vi "test main.vi"(8 "error in (no error)":errorcluster) -> (0 "error out":errorcluster)   [LabVIEW 2023]
uses:
  sequenceManagerWorker/sequenceManagerWorker.lvclass
  sequenceManagerWorker/ZE_Easy.Sequencer.lvlibp/Step/Step.lvclass
  f0be651f-cbc1-426a-b5fe-e5e117e5ce35.vi
  f17cfda4-eca7-44fe-abc0-9ba8470d04ab.vi
  ee86c54d-6899-49db-a6a4-df2ffb5378ed.vi
  d3de8112-106e-4eb0-9e2c-686bfc4be21a.vi
  7af16d0e-3bb2-44d1-b501-a320892e61ce.vi
  <vilib>/addons/_JKI Toolkits/Caraya/classes/Assert/Assert Equal Value and Type_Variant.vi
  <vilib>/addons/_JKI Toolkits/Caraya/classes/Assert/Assert Not Error.vi
  sequenceManagerWorker/ZE_Easy.Sequencer.lvlibp/Parameter/Parameter.lvclass
  <vilib>/addons/_JKI Toolkits/Caraya/classes/Test/Test.lvclass
  <vilib>/addons/_JKI Toolkits/Caraya/classes/Assert/Assert.lvclass
panel:
  # "Connector Pane"
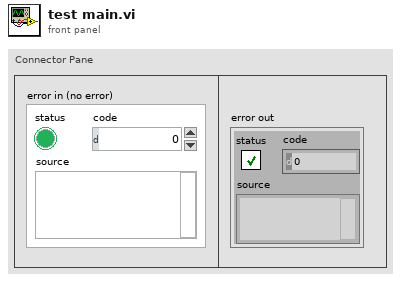
[diagram p1: front panel]
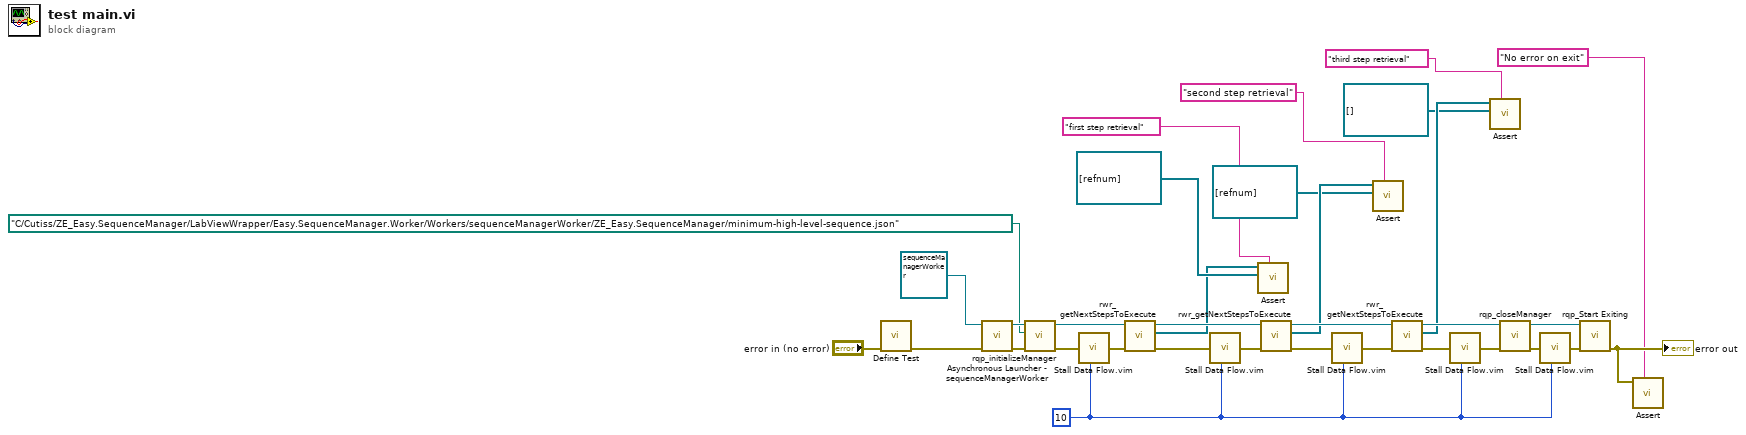
[diagram p0: block diagram]
diagram:
  w1 = u32 10 ("milliseconds to wait")
  n1 = call <vilib>:"Define Test.vi"("error in (no error)"="error in (no error)") -> ("error out"=w15:errorcluster)  [unwired: 9 in, 1 out]
  n2 = call "Asynchronous Launcher - sequenceManagerWorker.vi"("error in"=w15, "sequenceManagerWorker in"=refnum<class "sequenceManagerWorker.lvclass"> refnum) -> ("error out"=w31:errorcluster, "sequenceManagerWorker out"=w32:refnum<class "sequenceManagerWorker.lvclass">)  [unwired: 8 in]
  n3 = call "rqp_initializeManager.vi"("error in"=w31, "Path to JSON sequence file"=path "C:/Cutiss/ZE_Easy.SequenceManager/LabViewWrapper/Easy.SequenceManager.Worker/Workers/sequenceManagerWorker/ZE_Easy.SequenceManager/minimum-high-level-sequence.json", "sequenceManagerWorker in"=w32) -> ("error out"=w29:errorcluster, "dup sequenceManagerWorker out"=w30:refnum<class "sequenceManagerWorker.lvclass">)  [unwired: 6 in, 1 out]
  n4 = call "Stall Data Flow.vim"("value in"=w29, "milliseconds to wait"=w1) -> ("value out"=w21:errorcluster)  [unwired: 1 out]
  n5 = call "rwr_getNextStepsToExecute.vi"("error in"=w21, "sequenceManagerWorker in"=w30) -> ("error out"=w27:errorcluster, "StepsToExecuteInParallel"=w13:refnum<class "Step.lvclass">[], "dup sequenceManagerWorker out"=w28:refnum<class "sequenceManagerWorker.lvclass">)  [unwired: 6 in, 1 out]
  n6 = call "Stall Data Flow.vim"("value in"=w27, "milliseconds to wait"=w1) -> ("value out"=w20:errorcluster)  [unwired: 1 out]
  n7 = call-poly <vilib>:"Assert.vi"("Label"="first step retrieval" ("Label (VI Title)"), "Y"=refnum<class "Step.lvclass">[] [refnum] ("StepsToExecuteInParallel"), "X"=w13) -> ()  [unwired: 7 in, 2 out]
  n8 = call "rwr_getNextStepsToExecute.vi"("error in"=w20, "sequenceManagerWorker in"=w28) -> ("error out"=w25:errorcluster, "StepsToExecuteInParallel"=w11:refnum<class "Step.lvclass">[], "dup sequenceManagerWorker out"=w26:refnum<class "sequenceManagerWorker.lvclass">)  [unwired: 6 in, 1 out]
  n9 = call "Stall Data Flow.vim"("value in"=w25, "milliseconds to wait"=w1) -> ("value out"=w19:errorcluster)  [unwired: 1 out]
  n10 = call-poly <vilib>:"Assert.vi"("Label"="second step retrieval" ("Label (VI Title)"), "Y"=refnum<class "Step.lvclass">[] [refnum] ("StepsToExecuteInParallel 2"), "X"=w11) -> ()  [unwired: 7 in, 2 out]
  n11 = call "rwr_getNextStepsToExecute.vi"("error in"=w19, "sequenceManagerWorker in"=w26) -> ("error out"=w23:errorcluster, "StepsToExecuteInParallel"=w8:refnum<class "Step.lvclass">[], "dup sequenceManagerWorker out"=w24:refnum<class "sequenceManagerWorker.lvclass">)  [unwired: 6 in, 1 out]
  n12 = call "Stall Data Flow.vim"("value in"=w23, "milliseconds to wait"=w1) -> ("value out"=w18:errorcluster)  [unwired: 1 out]
  n13 = call-poly <vilib>:"Assert.vi"("Label"="third step retrieval" ("Label (VI Title)"), "Y"=refnum<class "Step.lvclass">[] [] ("StepsToExecuteInParallel 3"), "X"=w8) -> ()  [unwired: 7 in, 2 out]
  n14 = call "rqp_closeManager.vi"("error in"=w18, "sequenceManagerWorker in"=w24) -> ("error out"=w6:errorcluster, "dup sequenceManagerWorker out"=w5:refnum<class "sequenceManagerWorker.lvclass">)  [unwired: 7 in, 1 out]
  n15 = call "Stall Data Flow.vim"("value in"=w6, "milliseconds to wait"=w1) -> ("value out"=w2:errorcluster)  [unwired: 1 out]
  n16 = call "rqp_Start Exiting.vi"("error in"=w2, "sequenceManagerWorker in"=w5) -> ("error out"=w4:errorcluster)  [unwired: 7 in, 2 out]
  "error out" <- w4
  n17 = call-poly <vilib>:"Assert.vi"("Label"="No error on exit", "Not Error?"=w4) -> ()  [unwired: 8 in, 2 out]
